vi "process data.vi"(6 "state":T1=enum."Process data", 8 "error in (no error)":errorcluster, 10 "data input":dbl[](array[numeric])) -> (0 "error out":errorcluster, 1 "new interval":bool, 2 "averaged data":T2, 3 "total HRT":dbl, 5 "HRT (s)":dbl)   [LabVIEW 2019]
uses:
  data array with time.ctl
  data ave state.ctl
  data buffer cmd.ctl
  ini.ctl
  data channels.ctl
  state.ctl
  coag model data.ctl
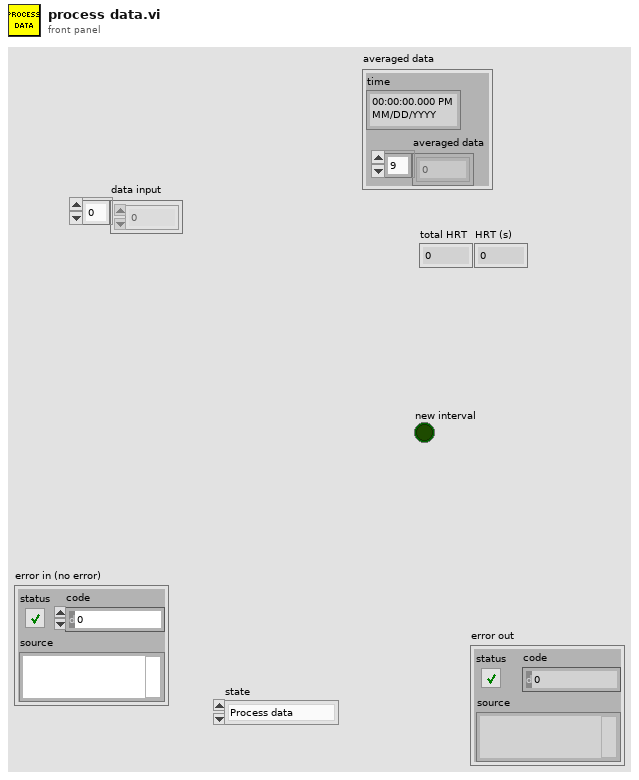
[diagram p1: front panel]
types:
  T1 = typedef "data ave state.ctl" = enum16{"Initialize", "Process data"}
  T2 = typedef "data array with time.ctl" = cluster{"time":timestamp, "averaged data":dbl[]}
  T3 = typedef "data buffer cmd.ctl" = enum16{"set buffer size", "write", "refill buffer", "read recent", "read all", "clear"}
  T4 = typedef "ini.ctl" = enum16{"write", "read"}
  T5 = typedef "coag model data.ctl" = cluster{"flow rate (L/s)":dbl, "Raw turbidity (NTU)":dbl, "floc sed turbidity (NTU)":dbl}
  T6 = typedef "state.ctl" = enum16{"Initialize", "Process data", "Close"}
  T7 = typedef "data channels.ctl" = enum16{"plant flow [L/s]", "Head Loss [m]", "sludge flow [L/s]", "UV 254", "raw [NTU]", "floc sed [NTU]", "clarified [NTU]", "filtered [NTU]"}
  T8 = typedef "setpoints.ctl" = cluster{"graph data interval (s)":sgl, "sludge flow [L/s]":dbl, "plant flow [L/s]":dbl, "Plant Flow PID ":cluster{"proportional gain (Kc)":dbl, "integral time (Ti, min)":dbl, "derivative time (Td, min)":dbl}, "Sludge PID ":cluster{"proportional gain (Kc)":dbl, "integral time (Ti, min)":dbl, "derivative time (Td, min)":dbl}, "backwash":T9, "Coagulant":T10}
  T9 = typedef "backwash.ctl" = cluster{"Filtered quality target [NTU]":dbl, "min filtration time [s]":dbl, "Ripen time [s]":dbl}
  T10 = typedef "coag.ctl" = cluster{"flocculator volume (L)":dbl, "clarifier volume (L)":dbl, "dose updates per HRT":u16, "target clarified turbidity (NTU)":dbl, "Coagulant mode":T11, "Coag dose [mg/L]":dbl, "pump mL/rev":dbl, "clarifier flow [L/s]":dbl, "min Coag dose [mg/L]":dbl, "max Coag dose [mg/L]":dbl, "Steps":u16, "HRT response delay":u32, "Ku*":dbl, "DOM coag demand [mg/L]":dbl, "min DOM coag demand [mg/L]":dbl, "max DOM coag demand [mg/L]":dbl}
  T11 = typedef "model type.ctl" = enum16{"manual", "ramp", "simple corrector"}
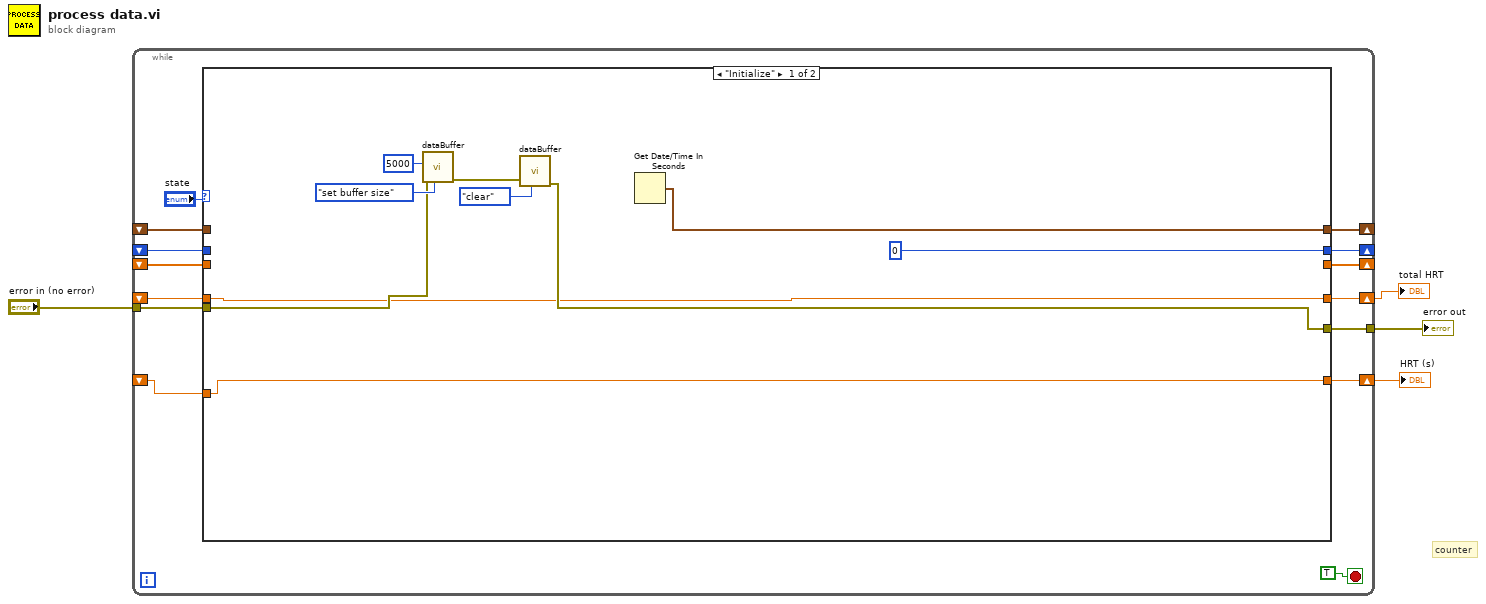
[diagram p0: block diagram]
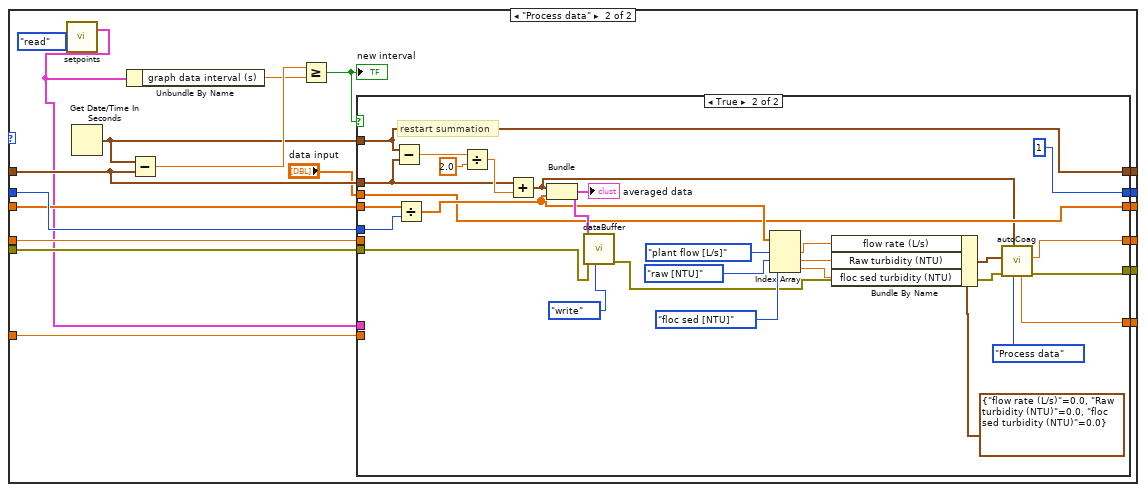
[diagram p2: hidden frame]
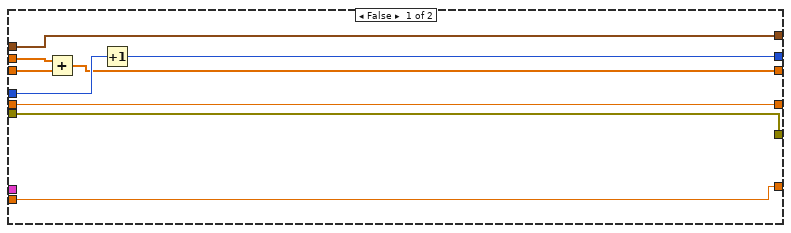
[diagram p3: hidden frame]
diagram:
  # "counter"
  n1 = while {
    shift-right: [w15] -> _
    shift-left: _ -> [w12]
    shift-right: [w17] -> _
    shift-left: _ -> [w16]
    shift-right: [w14] -> _
    shift-left: _ -> [w13]
    tunnel: "error in (no error)" -> [w10]
    tunnel: [w9] -> w3
    shift-right: [w8] -> w2
    shift-left: _ -> [w7]
    shift-right: [w6] -> w1
    shift-left: _ -> [w5]
    stop <- TRUE stop-if-true
    n2 = case shown="\"Initialize\"" "state" {
      tunnel: [0 w47] -> w17
      tunnel: w16 -> [_ w46]
      tunnel: [w28 w45] -> w15
      tunnel: [_ w44] -> w14
      tunnel: w13 -> [_ w43]
      tunnel: w12 -> [_ w42]
      tunnel: [w21 w35] -> w9
      tunnel: w10 -> [w22 w36]
      tunnel: [w20 w34] -> w8
      tunnel: w7 -> [w20 w33]
      tunnel: [w19 w30] -> w6
      tunnel: w5 -> [w19 w29]
      frame "Initialize" {
        n3 = call "dataBuffer.vi"("command"=data_buffer_cmd."set buffer size", "error in (no error)"=w22, "max array size"=u16 5000) -> ("error out"=w23:errorcluster)  [unwired: 3 in, 5 out]
        n4 = call "dataBuffer.vi"("command"=data_buffer_cmd."clear", "error in (no error)"=w23) -> ("error out"=w21:errorcluster)  [unwired: 4 in, 5 out]
        n5 = Get Date/Time In Seconds() -> (seconds since 1Jan1904=w28:timestamp)
      }
      frame "Process data" {
        n6 = call "setpoints.vi"("ini"=ini."read") -> ("Setpoints out"=w31:T8)  [unwired: 9 in, 1 out]
        n7 = Get Date/Time In Seconds() -> (seconds since 1Jan1904=w37:timestamp)
        n8 = Unbundle By Name(w31) -> ("graph data interval (s)"=w40:sgl)
        n9 = Subtract(x=w37, y=w42) -> (x-y=w41:dbl)
        n10 = Greater Or Equal?(x=w41, y=w40) -> (x >= y?=w39:bool)
        "new interval" <- w39
        n11 = case shown="True" w39 {
          tunnel: [w55 1] -> w47
          tunnel: w46 -> [w56 w77]
          tunnel: [w54 w76] -> w45
          tunnel: w37 -> [_ w76]
          tunnel: w42 -> [w54 w78]
          tunnel: [w52 w72] -> w44
          tunnel: w43 -> [w53 w82]
          tunnel: "data input" -> [w51 w72]
          tunnel: w36 -> [w50 w74]
          tunnel: [w50 w65] -> w35
          tunnel: w31 -> [_ _]
          tunnel: [w49 w64] -> w34
          tunnel: w33 -> [w49 _]
          tunnel: [w48 w57] -> w30
          tunnel: w29 -> [w48 _]
          frame False {
            n12 = Add(x=w51, y=w53) -> (x+y=w52:dbl[])
            n13 = Increment(x=w56) -> (x+1=w55:i32)
          }
          frame True {
            # "restart summation"
            n14 = Subtract(x=w76, y=w78) -> (x-y=w80:dbl)
            n15 = Divide(x=w82, y=w77) -> (x/y=w73:dbl[])
            n16 = Divide(x=w80, y=2.0) -> (x/y=w79:dbl)
            n17 = Add(x=w78, y=w79) -> (x+y=w67:timestamp)
            n18 = Bundle(w67, w73) -> (w75:cluster{timestamp, dbl[]})  [unwired: 1 in]
            "averaged data" <- w75
            n19 = call "dataBuffer.vi"("command"=data_buffer_cmd."write", "error in (no error)"=w74, "averaged data"=w75) -> ("error out"=w66:errorcluster)  [unwired: 3 in, 5 out]
            n20 = Index Array(array=w73, index #1=data_channels."plant flow [L/s]" ("channel"), index #2=data_channels."raw [NTU]" ("channel"), index #3=data_channels."floc sed [NTU]" ("channel")) -> (element #1=w63:dbl, element #2=w60:dbl, element #3=w59:dbl)
            n21 = Bundle By Name(cluster=T5 {"flow rate (L/s)"=0.0, "Raw turbidity (NTU)"=0.0, "floc sed turbidity (NTU)"=0.0} ("data input"), "flow rate (L/s)"=w63, "Raw turbidity (NTU)"=w60, "floc sed turbidity (NTU)"=w59) -> (w61:T5)
            n22 = call "autoCoag.vi"("state"=state."Process data", "current time"=w67, "error in (no error)"=w66, "data input"=w61) -> ("error out"=w65:errorcluster, "total HRT"=w64:dbl, "HRT (s)"=w57:dbl)  [unwired: 5 in]
          }
        }
      }
    }
  }
  "error out" <- w3
  "total HRT" <- w2
  "HRT (s)" <- w1
